vi "9215_fgv.vi"(7 "cmd":enum16{"config", "start", "read", "close"}(ring), 8 "error in":errorcluster caption="에러 입력", 10 "number of samples per channel":i32=-1 caption="채널당 샘플 개수", 11 "rate":dbl=100000.0 format="%0.2f") -> (0 "error out":errorcluster caption="에러 출력", 3 "data":waveform(dbl)[](array[waveform]) caption="데이터")   [LabVIEW 2013]
uses:
  <vilib>/DAQmx/read.llb/DAQmx Read.vi
  <vilib>/DAQmx/read.llb/DAQmx Read (Analog 1D Wfm NChan NSamp).vi
  <vilib>/DAQmx/create/channels.llb/DAQmx Create Channel (AI-Voltage-Basic).vi
  <vilib>/DAQmx/configure/timing.llb/DAQmx Timing (Sample Clock).vi
  <vilib>/DAQmx/miscellaneous.llb/DAQmx Fill In Error Info.vi
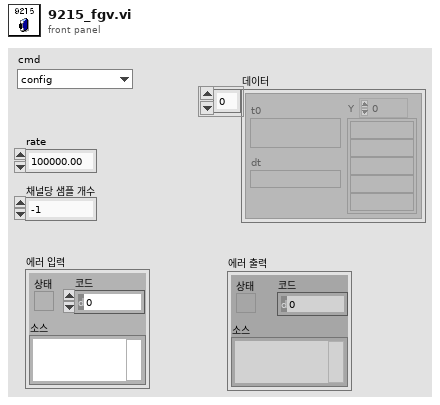
[diagram p1: front panel]
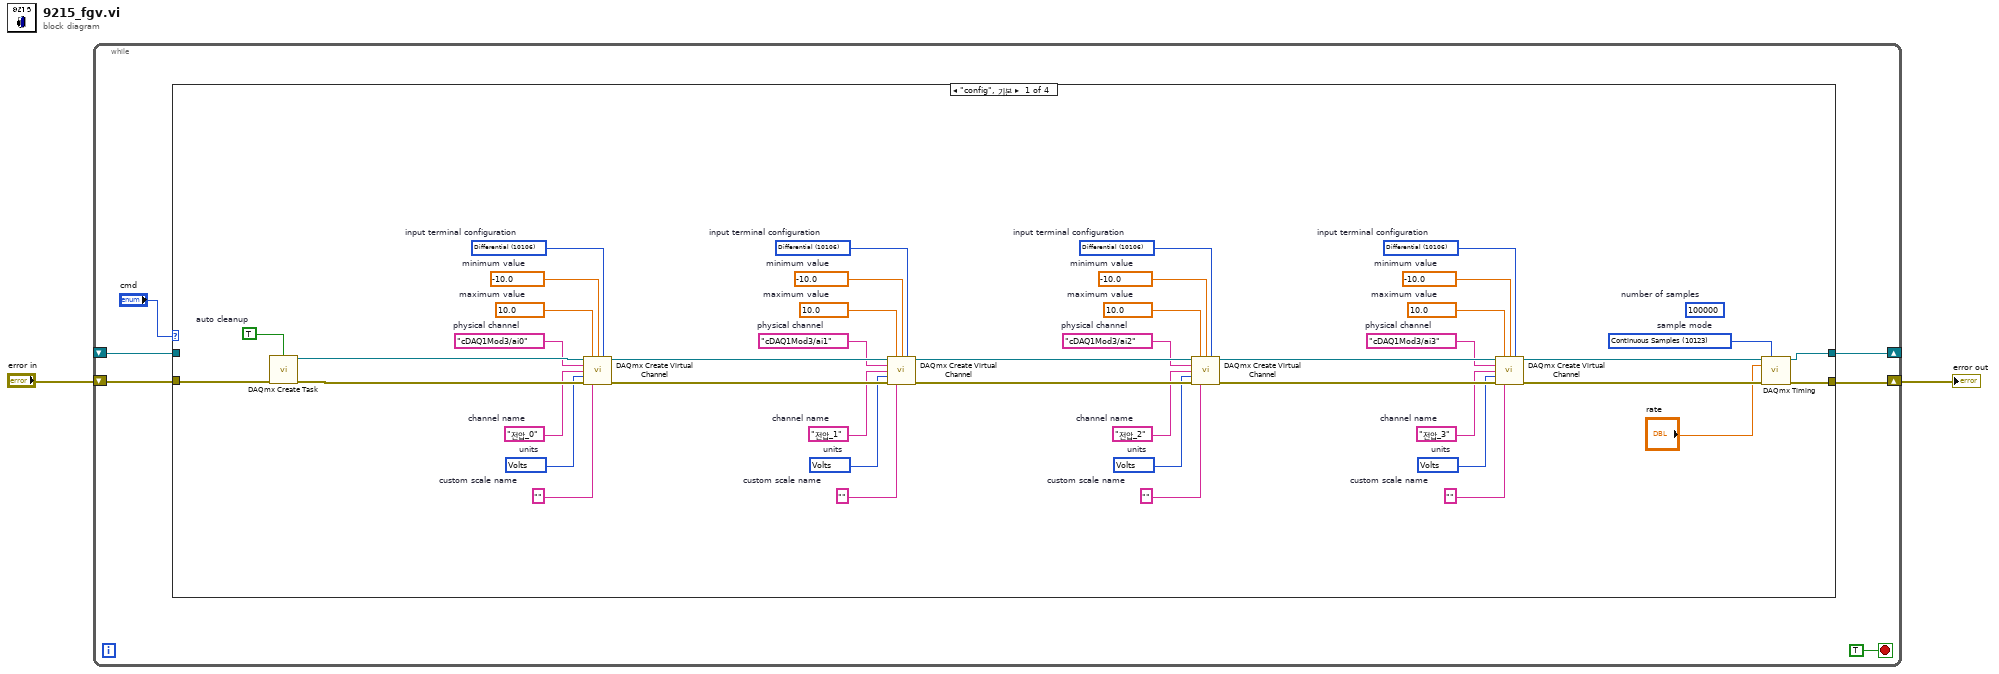
[diagram p0: block diagram]
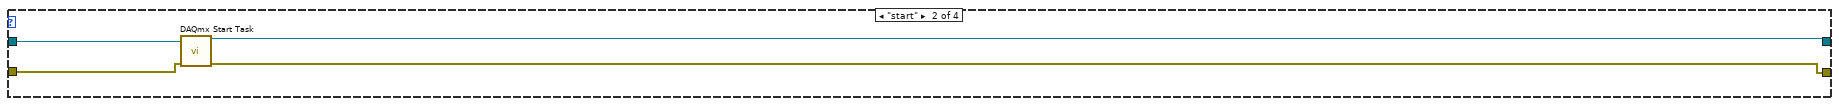
[diagram p2: hidden frame]
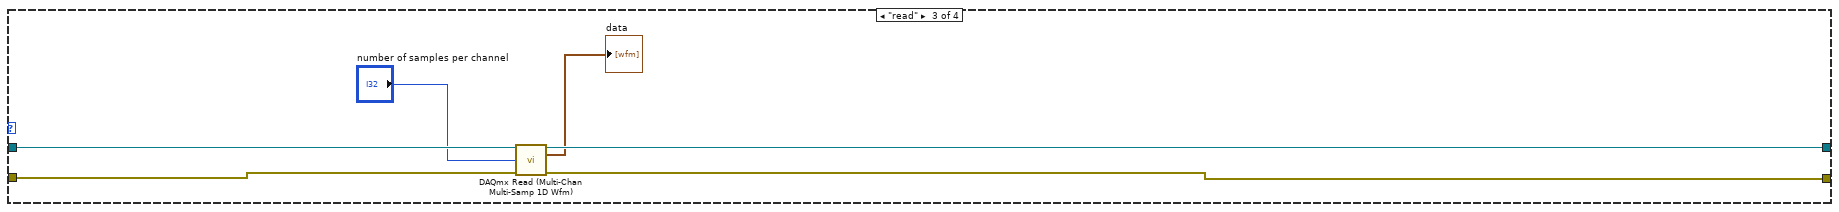
[diagram p3: hidden frame]
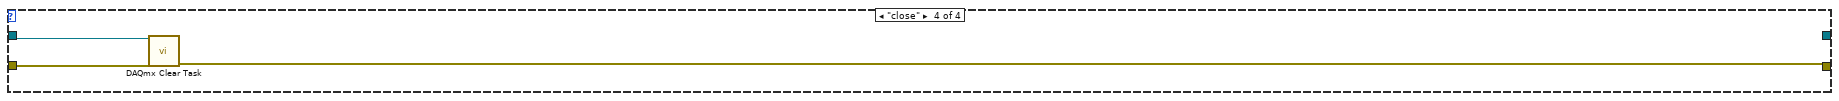
[diagram p4: hidden frame]
diagram:
  n1 = while {
    shift-right: [w7] -> w1
    shift-left: "error in" -> [w6]
    shift-right: [w5] -> _
    shift-left: _ -> [w3]
    stop <- TRUE stop-if-true
    n2 = case shown="\"config\", 기본" "cmd" {
      tunnel: [w11 w53 w60 w63] -> w7
      tunnel: w6 -> [w10 w56 w62 w65]
      tunnel: [w9 w54 w59 _] -> w5
      tunnel: w3 -> [_ w55 w61 w64]
      frame "config", Default {
        w12 = 10123 items=["Finite Samples"=10178, "Continuous Samples"=10123, "Hardware Timed Single Point"=12522]  # sample mode
        (unwired) 100000  # number of samples
        w15 = 10106 items=["default"=-1, "RSE"=10083, "NRSE"=10078, "Differential"=10106, "Pseudodifferential"=12529]  # input terminal configuration
        w16 = 10348 items=["Volts"=10348, "From Custom Scale"=10065]  # units
        w17 = "전압_3"  # channel name
        w19 = ""  # custom scale name
        w20 = -10.0  # minimum value
        w21 = 10.0  # maximum value
        w22 = "cDAQ1Mod3/ai3"  # physical channel
        w24 = 10106 items=["default"=-1, "RSE"=10083, "NRSE"=10078, "Differential"=10106, "Pseudodifferential"=12529]  # input terminal configuration
        w25 = 10348 items=["Volts"=10348, "From Custom Scale"=10065]  # units
        w26 = "전압_2"  # channel name
        w28 = ""  # custom scale name
        w29 = -10.0  # minimum value
        w30 = 10.0  # maximum value
        w31 = "cDAQ1Mod3/ai2"  # physical channel
        w33 = 10106 items=["default"=-1, "RSE"=10083, "NRSE"=10078, "Differential"=10106, "Pseudodifferential"=12529]  # input terminal configuration
        w34 = 10348 items=["Volts"=10348, "From Custom Scale"=10065]  # units
        w35 = "전압_1"  # channel name
        w37 = ""  # custom scale name
        w38 = -10.0  # minimum value
        w39 = 10.0  # maximum value
        w40 = "cDAQ1Mod3/ai1"  # physical channel
        w42 = 10106 items=["default"=-1, "RSE"=10083, "NRSE"=10078, "Differential"=10106, "Pseudodifferential"=12529]  # input terminal configuration
        w43 = 10348 items=["Volts"=10348, "From Custom Scale"=10065]  # units
        w44 = "전압_0"  # channel name
        w46 = ""  # custom scale name
        w47 = -10.0  # minimum value
        w48 = 10.0  # maximum value
        w49 = "cDAQ1Mod3/ai0"  # physical channel
        w51 = TRUE  # auto cleanup
        n3 = call <vilib>:"DAQmx Create Task.vi"("auto cleanup"=w51, "error in"=w10) -> ("task out"=w50:refnum<k21>, "error out"=w52:errorcluster)  [unwired: 12 in]
        n4 = call-poly <vilib>:"DAQmx Create Virtual Channel.vi"("task in"=w50, "maximum value"=w48, "minimum value"=w47, "input terminal configuration"=w42, "physical channels"=w49, "name to assign"=w44, "units"=w43, "error in"=w52, "custom scale name"=w46) -> ("task out"=w41:refnum<k21>, "error out"=w45:errorcluster)  [unwired: 5 in]
        n5 = call-poly <vilib>:"DAQmx Create Virtual Channel.vi"("task in"=w41, "maximum value"=w39, "minimum value"=w38, "input terminal configuration"=w33, "physical channels"=w40, "name to assign"=w35, "units"=w34, "error in"=w45, "custom scale name"=w37) -> ("task out"=w32:refnum<k21>, "error out"=w36:errorcluster)  [unwired: 5 in]
        n6 = call-poly <vilib>:"DAQmx Create Virtual Channel.vi"("task in"=w32, "maximum value"=w30, "minimum value"=w29, "input terminal configuration"=w24, "physical channels"=w31, "name to assign"=w26, "units"=w25, "error in"=w36, "custom scale name"=w28) -> ("task out"=w23:refnum<k21>, "error out"=w27:errorcluster)  [unwired: 5 in]
        n7 = call-poly <vilib>:"DAQmx Create Virtual Channel.vi"("task in"=w23, "maximum value"=w21, "minimum value"=w20, "input terminal configuration"=w15, "physical channels"=w22, "name to assign"=w17, "units"=w16, "error in"=w27, "custom scale name"=w19) -> ("task out"=w14:refnum<k21>, "error out"=w18:errorcluster)  [unwired: 5 in]
        n8 = call-poly <vilib>:"DAQmx Timing.vi"("task/channels in"=w14, "sample mode"=w12, "rate"="rate", "error in"=w18) -> ("task out"=w9:refnum<k21>, "error out"=w11:errorcluster)  [unwired: 10 in]
      }
      frame "start" {
        n9 = call <vilib>:"DAQmx Start Task.vi"("task/channels in"=w55, "error in"=w56) -> ("task out"=w54:refnum<k21>, "error out"=w53:errorcluster)  [unwired: 12 in]
      }
      frame "read" {
        n10 = call-poly "DAQmx Read (Multi-Chan Multi-Samp 1D Wfm).vi"("task/channels in"=w61, "number of samples per channel"="number of samples per channel", "error in"=w62) -> ("task out"=w59:refnum<k21>, "data"=→"data":waveform(dbl)[], "error out"=w60:errorcluster)  [unwired: 10 in]
      }
      frame "close" {
        n11 = call <vilib>:"DAQmx Clear Task.vi"("task in"=w64, "error in"=w65) -> ("error out"=w63:errorcluster)  [unwired: 13 in]
      }
    }
  }
  "error out" <- w1
